vi "Acquire_wp_nodt.vi"(0 "Ch Armed Reg":refnum<k21>="Register 1", 1 "Command FIFO":refnum<k21>, 3 "Circular Buffer Mem":refnum<k21>, 4 "circular buffer length":u32=300, 5 "FPGA I/O In":refnum<k21>="IO Module\\AI A0", 7 "channel on/off":bool, 9 "Trigger":i16=1500, 10 "Timing FIFO":refnum<k21>, 11 "Samples to Acquire":u32=100, 13 "Is Test Pulse?":bool, 14 "# of pretrigger":u32=15, 15 "timing":u64) -> ()   [LabVIEW 2012]
uses:
  <vilib>/rvi/DataTransferAndStorage/Container/Common/niFpgaContainerExecOnDevCompGetState.vi
  <vilib>/rvi/Memory/Memory_Emulation/nirvimemoryEmulationManagerCache_GetValue.vi
  <vilib>/rvi/Memory/Memory_Emulation/niFpgaMemoryEmulationValidateCache.vi
  <vilib>/rvi/DataTransferAndStorage/Container/Common/niFpgaContainerGetUniqueNameForEmu.vi
  <vilib>/rvi/Memory/Memory_Emulation/nirvimemoryEmulationManagerCache_InsertValue.vi
  <vilib>/rvi/eio/common/nirviEmuTemplateMethod_errors.vi
  <vilib>/rvi/Emulation/niFpgaSctlEmulationGetInTimedLoop.vi
  <vilib>/rvi/FIFO/Fifo_Resource/nirvififoEmulationSetSize.vi
  <vilib>/rvi/errors/niFpgaSetErrorForExecOnDevCompSimple.vi
  <vilib>/rvi/eio/common/nirviEmuReportErrorAndStop.vi
  <vilib>/rvi/Emulation/niFpgaSctlEmulationFifoFullMgr.vi
  <vilib>/rvi/Emulation/niFpgaSctlEmulationResourceMgr.vi
  <vilib>/rvi/interface/RandomDataEmulation/nirviRandomDataFPGAFIFO.vi
  <vilib>/rvi/interface/RandomDataEmulation/niFpgaRandomDataHandleErrors.vi
  <vilib>/rvi/DataTransferAndStorage/Container/XNode/niFpgaContainer.xnode
  <vilib>/rvi/DataTransferAndStorage/Register/Emulation/niFpgaRegisterEmulationRefIn.vi
  <vilib>/eio/EIONode/EIONode.xnode
  <vilib>/rvi/FIFO/Fifo_Resource/niFpgaFifoEmulationRefIn.vi
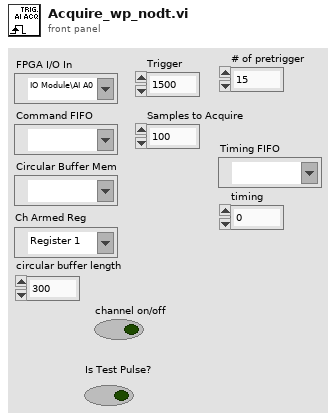
[diagram p1: front panel]
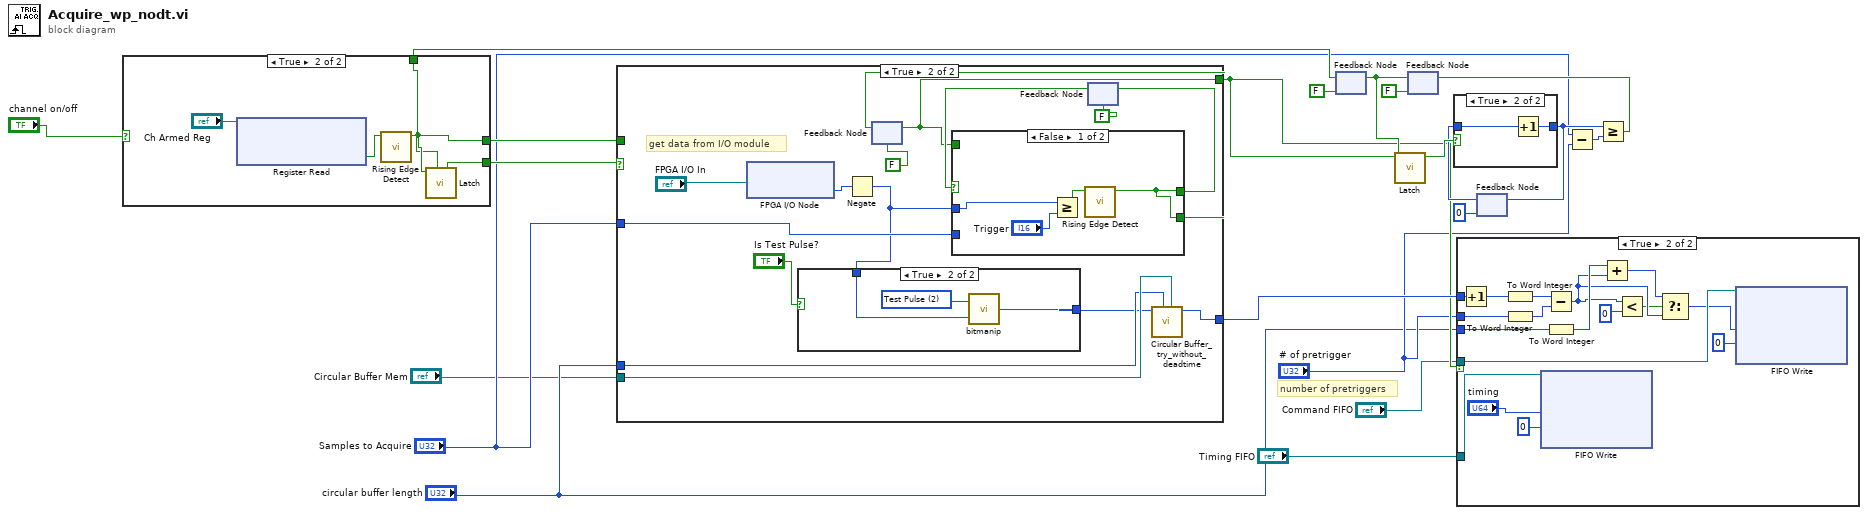
[diagram p0: block diagram]
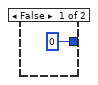
[diagram p3: hidden frame]
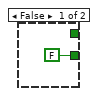
[diagram p4: hidden frame]
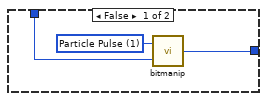
[diagram p6: hidden frame]
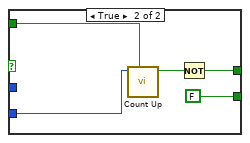
[diagram p7: hidden frame]
diagram:
  # "number of pretriggers"
  n1 = feedback #1(FALSE) -> (w16:bool)
  n2 = case shown="True" "channel on/off" {
    tunnel: [FALSE ("Output") w26] -> w21
    tunnel: [_ w27] -> w20
    tunnel: w16 -> [_ w25]
    frame False {
    }
    frame True {
      n3 = xnode ("Register Read")("Register In"="Ch Armed Reg") -> ("Data"=w23:bool)  [unwired: 1 out]
      n4 = call "Rising Edge Detect.vi"("Input"=w23) -> ("Rising Edge"=w27:bool)  [unwired: 10 in]
      n5 = call "Latch.vi"("Reset"=w25, "Input"=w27) -> ("Output"=w26:bool)  [unwired: 9 in]
    }
  }
  n6 = case shown="True" w21 {
    tunnel: "Circular Buffer Mem" -> [_ w42]
    tunnel: "circular buffer length" -> [_ w38]
    tunnel: [_ w41] -> w19
    tunnel: w20 -> [_ _]
    tunnel: "Samples to Acquire" -> [_ w37]
    tunnel: [_ w33] -> w8
    frame False {
    }
    frame True {
      # "get data from I/O module"
      n7 = xnode "FPGA I/O Node"("FPGA I/O In"="FPGA I/O In") -> ("I/O Item"=w29:i16)  [unwired: 1 out]
      n8 = Negate(x=w29) -> (-x=w28:i16)
      n9 = case shown="True" "Is Test Pulse?" {
        tunnel: w28 -> [w44 w47]
        tunnel: [w43 w46] -> w31
        frame False {
          w45 = u16 1 items=["Header Information", "Particle Pulse", "Test Pulse"] ("Pulse Type")
          n10 = call "bitmanip.vi"("Pulse Type"=w45, "Integer to be written"=w44) -> ("Integer Written"=w43:i16)  [unwired: 2 in]
        }
        frame True {
          w48 = u16 2 items=["Header Information", "Particle Pulse", "Test Pulse"] ("Pulse Type")
          n11 = call "bitmanip.vi"("Pulse Type"=w48, "Integer to be written"=w47) -> ("Integer Written"=w46:i16)  [unwired: 2 in]
        }
      }
      n12 = feedback #2(FALSE) -> (w33:bool)
      n13 = feedback #3(FALSE) -> (w36:bool)
      n14 = case shown="False" w36 {
        tunnel: w28 -> [w52 _]
        tunnel: w37 -> [_ w57]
        tunnel: w33 -> [_ w56]
        tunnel: [w50 w54] -> w35
        tunnel: [w50 FALSE] -> w34
        frame False {
          n15 = Greater Or Equal?(x=w52, y="Trigger") -> (x >= y?=w51:bool)
          n16 = call "Rising Edge Detect.vi"("Input"=w51) -> ("Rising Edge"=w50:bool)  [unwired: 10 in]
        }
        frame True {
          n17 = call "Count Up.vi"("Reset?"=w56, "goal"=w57) -> ("Count Met"=w55:bool)  [unwired: 8 in, 1 out]
          n18 = Not(x=w55) -> (.not. x?=w54:bool)
        }
      }
      n19 = feedback-in #2(w34) -> ()
      n20 = feedback-in #3(w35) -> ()
      n21 = call "Circular Buffer_try_without_deadtime.vi"("Refnum in"=w42, "circular buffer length"=w38, "Data"=w31) -> ("Address"=w41:u16)  [unwired: 8 in]
    }
  }
  n22 = feedback #4(FALSE) -> (w14:bool)
  n23 = feedback-in #1(w14) -> ()
  n24 = call "Latch.vi"("Reset"=w14, "Input"=w8) -> ("Output"=w12:bool)  [unwired: 9 in]
  n25 = case shown="True" w8 {
    tunnel: "Command FIFO" -> [_ w74]
    tunnel: "Timing FIFO" -> [_ w73]
    tunnel: w19 -> [_ w62]
    tunnel: "circular buffer length" -> [_ w60]
    tunnel: "# of pretrigger" -> [_ w59]
    frame False {
    }
    frame True {
      n26 = Increment(x=w62) -> (x+1=w68:u16)
      n27 = To Word Integer(number=w68) -> (16bit integer=w69:i16)
      n28 = To Word Integer(number=w59) -> (16bit integer=w70:i16)
      n29 = xnode ("FIFO Write")("Element"="timing", "Timeout"=0, "FIFO In"=w73) -> ()  [unwired: 2 out]
      n30 = Subtract(x=w69, y=w70) -> (x-y=w66:i16)
      n31 = To Word Integer(number=w60) -> (16bit integer=w67:i16)
      n32 = Add(x=w67, y=w66) -> (x+y=w65:i16)
      n33 = Less?(x=w66, y=i16 0) -> (x < y?=w63:bool)
      n34 = Select(t=w65, s=w63, f=w66) -> (s? t:f=w61:i16)
      n35 = xnode ("FIFO Write")("Element"=w61, "Timeout"=0, "FIFO In"=w74) -> ()  [unwired: 2 out]
    }
  }
  n36 = feedback #5(u32 0) -> (w11:u32)
  n37 = case shown="True" w12 {
    tunnel: w11 -> [_ w77]
    tunnel: [i16 0 w76] -> w9
    frame False {
    }
    frame True {
      n38 = Increment(x=w77) -> (x+1=w76:u32)
    }
  }
  n39 = feedback-in #5(w9) -> ()
  n40 = Subtract(x="Samples to Acquire", y="# of pretrigger") -> (x-y=w10:u32)
  n41 = Greater Or Equal?(x=w9, y=w10) -> (x >= y?=w15:bool)
  n42 = feedback-in #4(w15) -> ()
